vi "Controller Initialize Configuration.vi"(8 "error in (no error)":errorcluster, 11 "FOFB Configuration":T1) -> (0 "error out":errorcluster, 3 "FOFB Configuration":T1)   [LabVIEW 2011, in "Controller VIs.lvlib"]
uses:
  Controller VIs.lvlib
  Types Definitions/Type FOFB Configuration.ctl
  Types Definitions/Type FOFB Parameters.ctl
  Types Definitions/Type Network Configuration.ctl
  Types Definitions/Type FA Configuration.ctl
  Types Definitions/Type Acquisition Network Configuration.ctl
  Types Definitions/Type Actuation Network Configuration.ctl
  Types Definitions/Type Control FOFB Configuration Out.ctl
  Types Definitions/Type Operation Mode State.ctl
  Types Definitions/Type Control FOFB Configuration In.ctl
  Controller Global Variables/LNLS Control FOFB Configuration Out.vi
  Controller Global Variables/LNLS Control FOFB Configuration In.vi
  Type Definitions.lvlib
  Controller Global Variables.lvlib
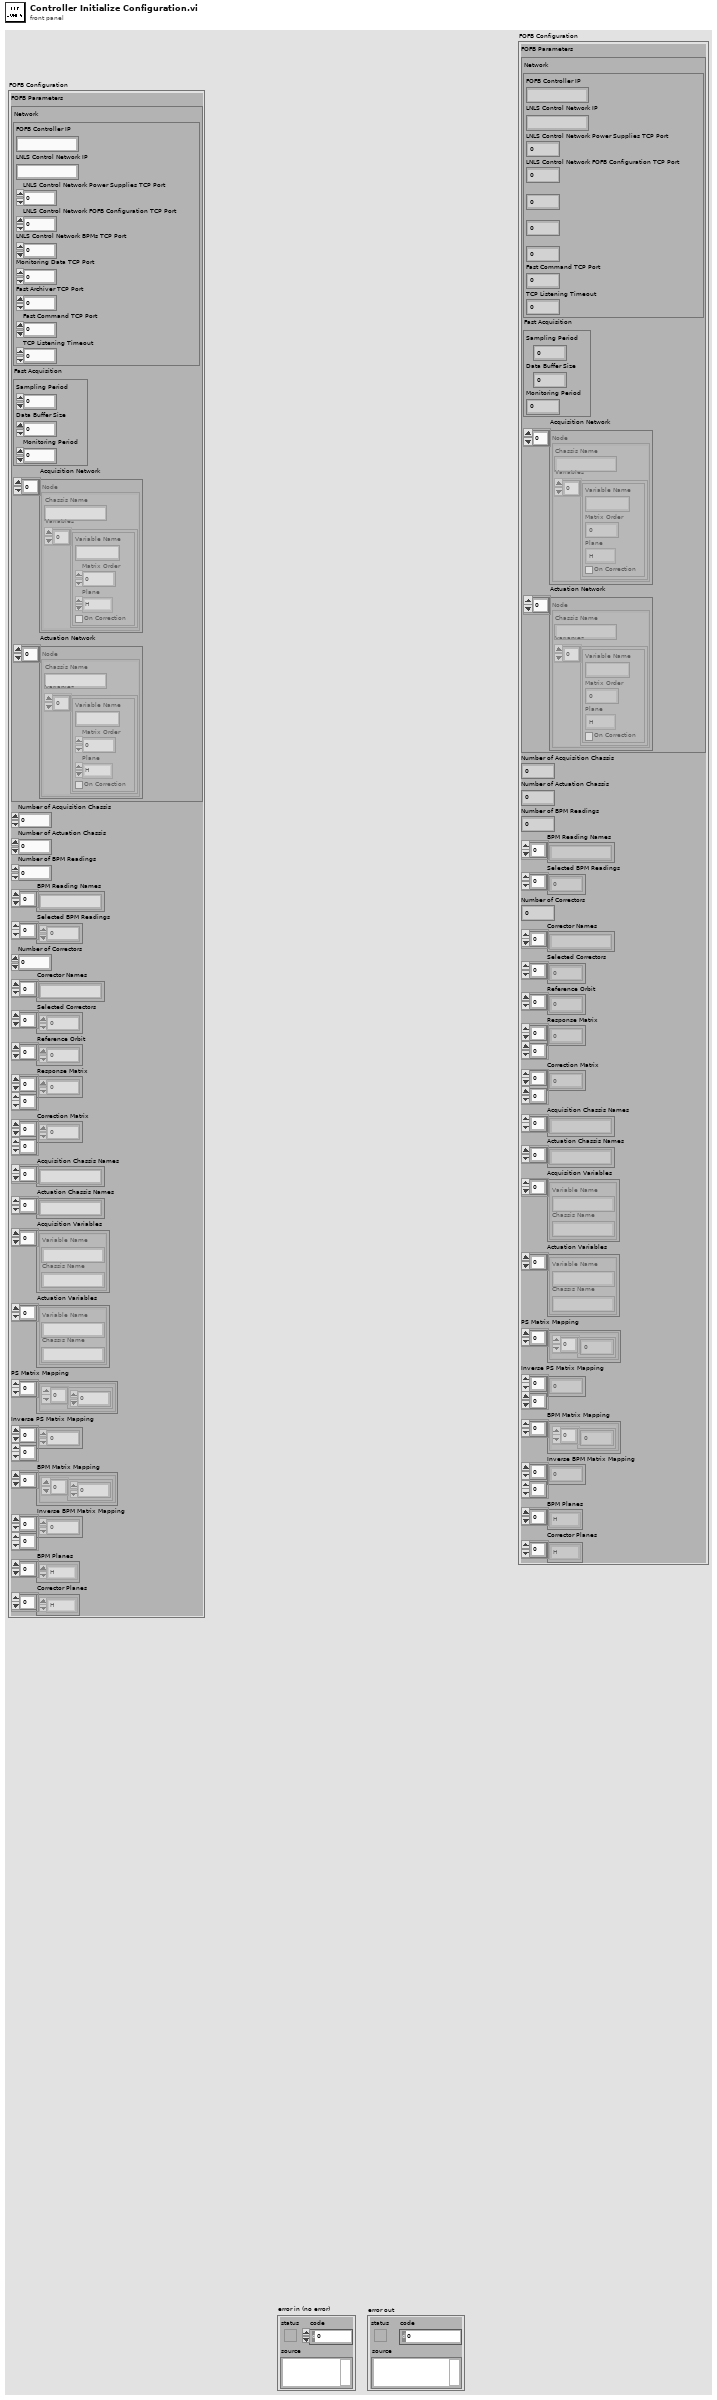
[diagram p1: front panel]
types:
  T1 = typedef "Type Definitions.lvlib/Type FOFB Configuration.ctl" = cluster{"FOFB Parameters":T2, "Number of Acquisition Chassis":i32, "Number of Actuation Chassis":i32, "Number of BPM Readings":i32, "BPM Reading Names":string[], "Selected BPM Readings":u32[], "Number of Correctors":i32, "Corrector Names":string[], "Selected Correctors":u32[], "Reference Orbit":dbl[], "Response Matrix":dbl[][], "Correction Matrix":dbl[][], "Acquisition Chassis Names":string[], "Actuation Chassis Names":string[], "Acquisition Variables":cluster{"Variable Name":string, "Chassis Name":string}[], "Actuation Variables":cluster{"Variable Name":string, "Chassis Name":string}[], "PS Matrix Mapping":cluster{u32[]}[], "Inverse PS Matrix Mapping":u32[][], "BPM Matrix Mapping":cluster{u32[]}[], "Inverse BPM Matrix Mapping":u32[][], "BPM Planes":enum8{"H", "V"}[], "Corrector Planes":enum8{"H", "V"}[]}
  T2 = typedef "Type Definitions.lvlib/Type FOFB Parameters.ctl" = cluster{"Network":T3, "Fast Acquisition":T4, "Acquisition Network":T5, "Actuation Network":T6}
  T3 = typedef "Type Definitions.lvlib/Type Network Configuration.ctl" = cluster{"FOFB Controller IP":string, "LNLS Control Network IP":string, "LNLS Control Network Power Supplies TCP Port":u16, "LNLS Control Network FOFB Configuration TCP Port":u16, "LNLS Control Network BPMs TCP Port":u16, "Monitoring Data TCP Port":u16, "Fast Archiver TCP Port":u16, "Fast Command TCP Port":u16, "TCP Listening Timeout":i32}
  T4 = typedef "Type Definitions.lvlib/Type FA Configuration.ctl" = cluster{"Sampling Period":u32, "Data Buffer Size":u32, "Monitoring Period":u32}
  T5 = typedef "Type Definitions.lvlib/Type Acquisition Network Configuration.ctl" = cluster{"Chassis Name":string, "Variables":cluster{"Variable Name":string, "Matrix Order":u32, "Plane":enum8{"H", "V"}, "On Correction":bool}[]}[]
  T6 = typedef "Type Definitions.lvlib/Type Actuation Network Configuration.ctl" = cluster{"Chassis Name":string, "Variables":cluster{"Variable Name":string, "Matrix Order":u32, "Plane":enum8{"H", "V"}, "On Correction":bool}[]}[]
  T7 = typedef "Type Definitions.lvlib/Type Control FOFB Configuration In.ctl" = cluster{"Status":u16, "Operation Mode":T8, "Horizontal Gain":sgl, "Vertical Gain":sgl, "PID Horizontal Integral Time":sgl, "PID Vertical Integral Time":sgl, "PID Horizontal Derivative Time":sgl, "PID Vertical Derivative Time":sgl, "Fast Command Enabled":bool}
  T8 = typedef "Type Definitions.lvlib/Type Operation Mode State.ctl" = enum8{"Idle Mode", "Manual Mode", "FOFB Mode"}
  T9 = typedef "Type Definitions.lvlib/Type Control FOFB Configuration Out.ctl" = cluster{"Status":u16, "Operation Mode":T8, "Horizontal Gain":sgl, "Vertical Gain":sgl, "PID Horizontal Integral Time":sgl, "PID Vertical Integral Time":sgl, "PID Horizontal Derivative Time":sgl, "PID Vertical Derivative Time":sgl, "Fast Command Enabled":bool, "RMS Horizontal Distortion":dbl, "RMS Vertical Distortion":dbl, "Timestamp":dbl}
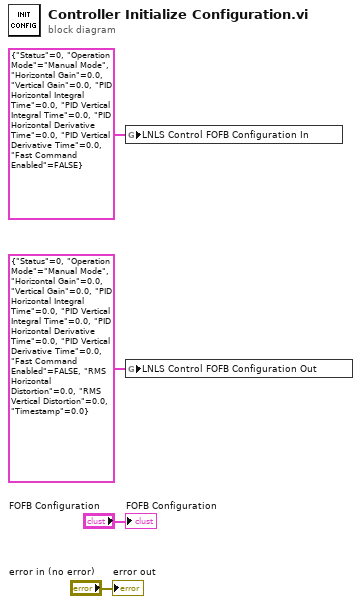
[diagram p0: block diagram]
diagram:
  n1 = global write "LNLS Control FOFB Configuration In.vi" "LNLS Control FOFB Configuration In"(T7 {"Status"=0, "Operation Mode"=enum."Manual Mode", "Horizontal Gain"=0.0, "Vertical Gain"=0.0, "PID Horizontal Integral Time"=0.0, "PID Vertical Integral Time"=0.0, "PID Horizontal Derivative Time"=0.0, "PID Vertical Derivative Time"=0.0, "Fast Command Enabled"=FALSE} ("LNLS Control FOFB Configuration In")) -> ()
  n2 = global write "LNLS Control FOFB Configuration Out.vi" "LNLS Control FOFB Configuration Out"(T9 {"Status"=0, "Operation Mode"=enum."Manual Mode", "Horizontal Gain"=0.0, "Vertical Gain"=0.0, "PID Horizontal Integral Time"=0.0, "PID Vertical Integral Time"=0.0, "PID Horizontal Derivative Time"=0.0, "PID Vertical Derivative Time"=0.0, "Fast Command Enabled"=FALSE, "RMS Horizontal Distortion"=0.0, "RMS Vertical Distortion"=0.0, "Timestamp"=0.0} ("LNLS Control FOFB Configuration Out")) -> ()
  "FOFB Configuration" <- "FOFB Configuration"
  "error out" <- "error in (no error)"
